vi "pmu_Frequency Interpolator.vi"(5 "reset? (F)":bool, 6 "reported time":dbl, 8 "error in (no error)":errorcluster, 9 "PMU system info in":refnum<class "PMU System Info.lvclass">, 10 "timestamps":dbl[](array[numeric]), 11 "frequencies":dbl[](array[numeric]) format="%_10g") -> (0 "error out":errorcluster, 1 "PMU system info out":refnum<class "PMU System Info.lvclass">, 2 "df/dt":sgl, 3 "frequency":sgl format="%_10g")   [LabVIEW 2013, in "NI_EP_PMU.lvlib"]
uses:
  <vilib>/addons/Electrical Power/PMU/NI_EP_PMU.lvlib
  <vilib>/addons/Electrical Power/PMU/Common/Classes/PMU System Info/PMU System Info.lvclass
  <vilib>/Analysis/NI_AALPro.lvlib
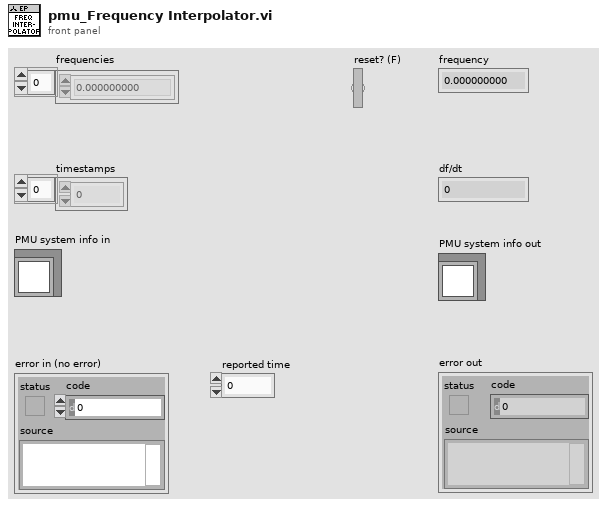
[diagram p1: front panel]
types:
  T1 = typedef "NI_EP_PMU.lvlib/pmu_ROCOF Detector Settings.ctl" = cluster{"ROCOF window width":i32}
  T2 = typedef "NI_EP_PMU.lvlib/pmu_Frequency Detector Settings.ctl" = cluster{"frequency window width":i32}
  T3 = typedef "NI_EP_PMU.lvlib/pmu_CFG Class.ctl" = cluster{"station name":string, "PMU ID":u16, "time base":u32, "nominal frequency":enum16{"50 Hz", "60 Hz"}, "reporting rate":i16, "phasor number":u16, "analog number":u16, "digital number":u16, "channel names":string[], "phasor units":u32[], "analog units":u32[], "digital units":u32[], "data format":u16, "number of PMUs":u16}
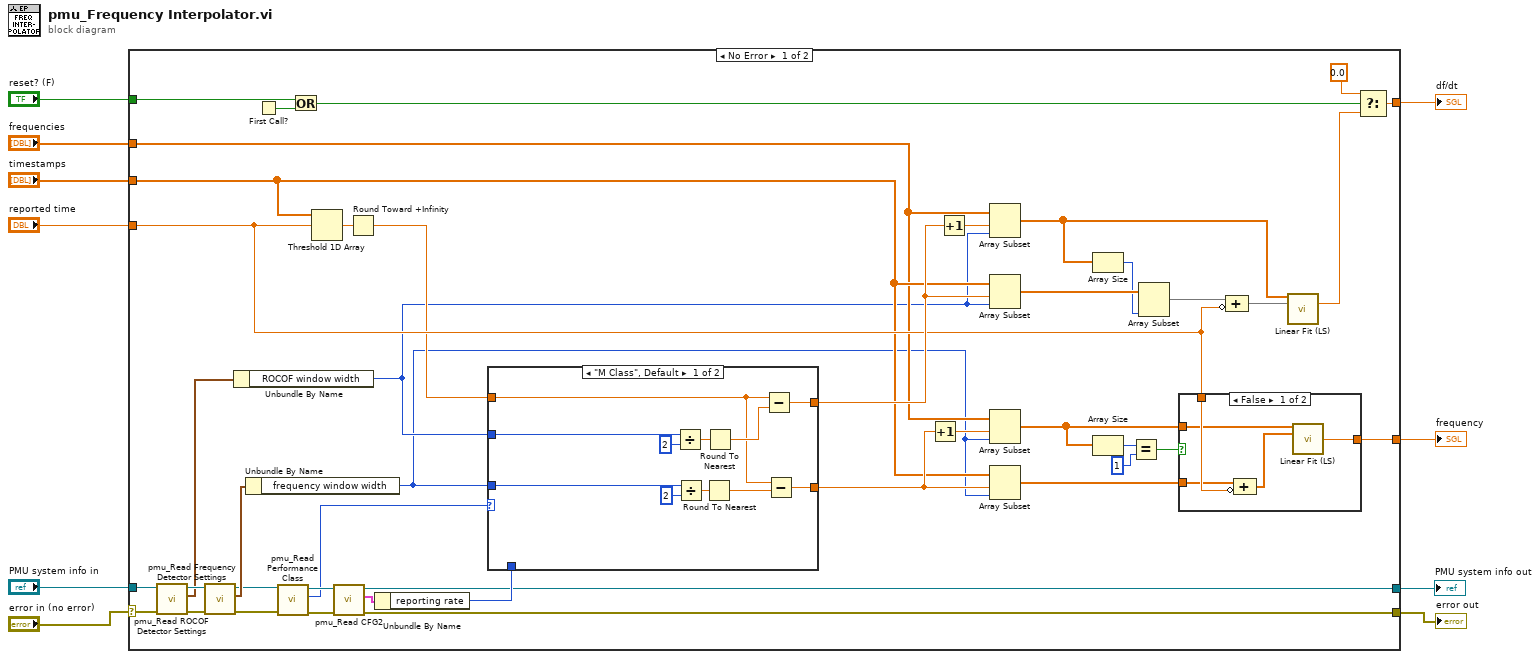
[diagram p0: block diagram]
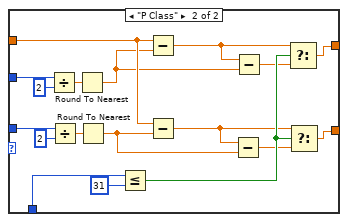
[diagram p2: hidden frame]
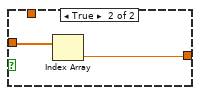
[diagram p3: hidden frame]
diagram:
  n1 = case shown="No Error" "error in (no error)" {
    selector: "error in (no error)" -> [w13 w90]
    tunnel: "reset? (F)" -> [w51 _]
    tunnel: [w48 _] -> w9
    tunnel: "reported time" -> [w42 _]
    tunnel: "timestamps" -> [w41 _]
    tunnel: [w40 _] -> w6
    tunnel: "frequencies" -> [w33 _]
    tunnel: "PMU system info in" -> [w21 _]
    tunnel: [w12 w90] -> w2
    tunnel: [w11 _] -> w1
    frame No Error {
      n2 = call <vilib>:"pmu_Read ROCOF Detector Settings.vi"("error in (no error)"=w13, "system info in"=w21) -> ("error out"=w26:errorcluster, "ROCOF detector settings"=w24:T1, "system info out"=w25:refnum<class "PMU System Info.lvclass">)  [unwired: 7 in]
      n3 = call <vilib>:"pmu_Read Frequency Detector Settings.vi"("error in (no error)"=w26, "system info in"=w25) -> ("error out"=w20:errorcluster, "frequency detector settings"=w27:T2, "system info out"=w19:refnum<class "PMU System Info.lvclass">)  [unwired: 7 in]
      n4 = Unbundle By Name(w24) -> ("ROCOF window width"=w23:i32)
      n5 = Unbundle By Name(w27) -> ("frequency window width"=w14:i32)
      n6 = First Call?() -> (First Call?: T/F=w52:bool)
      n7 = call <vilib>:"pmu_Read Performance Class.vi"("error in (no error)"=w20, "system info in"=w19) -> ("error out"=w17:errorcluster, "performance class"=w16:enum8{"M Class", "P Class"}, "system info out"=w18:refnum<class "PMU System Info.lvclass">)  [unwired: 7 in]
      n8 = Or(x=w51, y=w52) -> (x .or. y?=w50:bool)
      n9 = Threshold 1D Array(2:w42, 3:w41) -> (0:w47:dbl)  [unwired: 1 in]
      n10 = call <vilib>:"pmu_Read CFG2.vi"("error in (no error)"=w17, "system info in"=w18) -> ("error out"=w12:errorcluster, "CFG-2"=w22:T3, "system info out"=w11:refnum<class "PMU System Info.lvclass">)  [unwired: 7 in]
      n11 = Round Toward +Infinity(x=w47) -> (ceil(x): smallest int >= x=w32:dbl)
      n12 = Unbundle By Name(w22) -> ("reporting rate"=w15:i16)
      n13 = case shown="\"M Class\", Default" w16 {
        tunnel: [w63 w79] -> w49
        tunnel: [w59 w78] -> w46
        tunnel: w32 -> [w56 w70]
        tunnel: w14 -> [w55 w71]
        tunnel: w23 -> [w54 w74]
        tunnel: w15 -> [_ w77]
        frame "M Class", Default {
          n14 = Divide(x=w54, y=2) -> (x/y=w62:dbl)
          n15 = Divide(x=w55, y=2) -> (x/y=w60:dbl)
          n16 = Round To Nearest(number=w60) -> (nearest integer value=w57:dbl)
          n17 = Round To Nearest(number=w62) -> (nearest integer value=w58:dbl)
          n18 = Subtract(x=w56, y=w58) -> (x-y=w63:dbl)
          n19 = Subtract(x=w56, y=w57) -> (x-y=w59:dbl)
        }
        frame "P Class" {
          n20 = Divide(x=w74, y=2) -> (x/y=w75:dbl)
          n21 = Divide(x=w71, y=2) -> (x/y=w73:dbl)
          n22 = Round To Nearest(number=w75) -> (nearest integer value=w69:dbl)
          n23 = Round To Nearest(number=w73) -> (nearest integer value=w65:dbl)
          n24 = Less Or Equal?(x=w77, y=i16 31) -> (x <= y?=w81:bool)
          n25 = Subtract(x=w70, y=w69) -> (x-y=w68:dbl)
          n26 = Subtract(x=w70, y=w65) -> (x-y=w66:dbl)
          n27 = Subtract(x=w66, y=w65) -> (x-y=w67:dbl)
          n28 = Subtract(x=w68, y=w69) -> (x-y=w80:dbl)
          n29 = Select(t=w68, s=w81, f=w80) -> (s? t:f=w79:dbl)
          n30 = Select(t=w66, s=w81, f=w67) -> (s? t:f=w78:dbl)
        }
      }
      n31 = Increment(x=w46) -> (x+1=w43:dbl)
      n32 = Increment(x=w49) -> (x+1=w45:dbl)
      n33 = Array Subset(array=w33, index=w45, length=w23) -> (w36:dbl[])
      n34 = Array Subset(array=w41, index=w49, length=w23) -> (w37:dbl[])
      n35 = Array Subset(array=w33, index=w43, length=w14) -> (w31:dbl[])
      n36 = Array Subset(array=w41, index=w46, length=w14) -> (w38:dbl[])
      n37 = Array Size(array=w36) -> (size(s)=w34:i32)
      n38 = Array Size(array=w31) -> (size(s)=w30:i32)
      n39 = Equal?(x=w30, y=1) -> (x = y?=w28:bool)
      n40 = Array Subset(array=w37, length=w34) -> (w35:dbl[])  [unwired: 1 in]
      n41 = case shown="False" w28 {
        tunnel: w42 -> [w86 _]
        tunnel: [w85 w88] -> w40
        tunnel: w38 -> [w84 _]
        tunnel: w31 -> [w83 w89]
        frame False {
          n42 = Compound Arithmetic op=ADD(w84, invert w86) -> (w87:dbl[])
          n43 = call <vilib>:"Linear Fit (LS).vi"("Y"=w83, "X"=w87) -> ("intercept"=w85:dbl)  [unwired: 1 in, 12 out]
        }
        frame True {
          n44 = Index Array(array=w89) -> (element=w88:dbl)  [unwired: 1 in]
        }
      }
      n45 = Compound Arithmetic op=ADD(w35, invert w42) -> (w44:dbl[])
      n46 = call <vilib>:"Linear Fit (LS).vi"("Y"=w36, "X"=w44) -> ("slope"=w39:dbl)  [unwired: 1 in, 12 out]
      n47 = Select(t=0.0, s=w50, f=w39) -> (s? t:f=w48:dbl)
    }
    frame Error {
    }
  }
  "frequency" <- w6
  "df/dt" <- w9
  "error out" <- w2
  "PMU system info out" <- w1
